vi "VISA write.vi"(8 "error in (no error)":errorcluster, 10 "stringtowrite":string, 11 "Cobolt in":refnum<class "Cobolt.lvclass">) -> (0 "error out":errorcluster, 3 "Cobolt out":refnum<class "Cobolt.lvclass">)   [LabVIEW 2012, in "Cobolt.lvclass"]
uses:
  Cobolt.lvclass
  Cobolt.lvclass/Cobolt.ctl
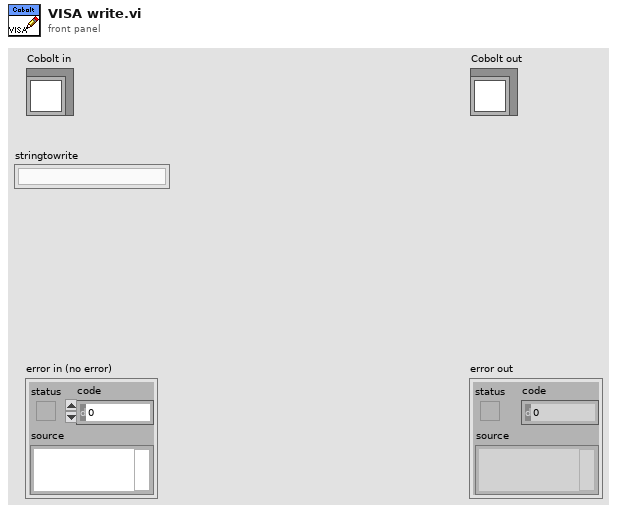
[diagram p1: front panel]
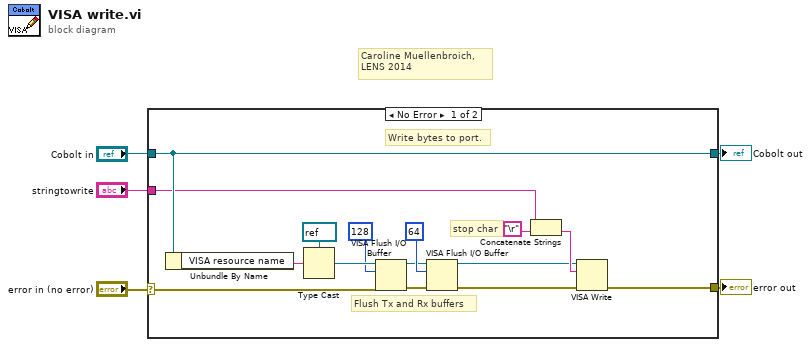
[diagram p0: block diagram]
diagram:
  # "Caroline Muellenbroich, \nLENS 2014"
  n1 = case shown="No Error" "error in (no error)" {
    selector: "error in (no error)" -> [w12 w22]
    tunnel: [w15 w22] -> w4
    tunnel: [w16 w21] -> w2
    tunnel: "Cobolt in" -> [w16 w21]
    tunnel: "stringtowrite" -> [w10 _]
    frame No Error {
      # "stop char"
      # "Flush Tx and Rx buffers"
      # "Write bytes to port."
      n2 = Unbundle By Name(w16) -> ("VISA resource name"=w20:string)
      n3 = Type Cast(type=refnum<visa-resource-name> refnum ("VISA resource name"), x=w20) -> (*(type *) &x=w14:refnum<visa-resource-name>)
      n4 = VISA Flush I/O Buffer(VISA resource name=w14, mask (16)=u16 128, error in (no error)=w12) -> (VISA resource name out=w7:refnum<visa-resource-name>, error out=w6:errorcluster)
      n5 = VISA Flush I/O Buffer(VISA resource name=w7, mask (16)=u16 64, error in (no error)=w6) -> (VISA resource name out=w13:refnum<visa-resource-name>, error out=w11:errorcluster)
      n6 = Concatenate Strings(w10, "\r") -> (w18:string)
      n7 = VISA Write(VISA resource name=w13, write buffer=w18, error in (no error)=w11) -> (error out=w15:errorcluster)  [unwired: 2 out]
    }
    frame Error {
    }
  }
  "error out" <- w4
  "Cobolt out" <- w2
